vi "GetLastChar.vi"(10 "String":string) -> (2 "String 2":string)   [LabVIEW 2016]
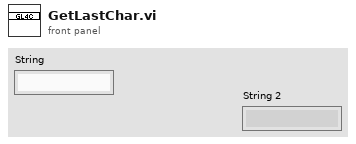
[diagram p1: front panel]
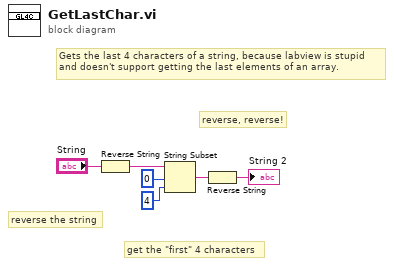
[diagram p0: block diagram]
diagram:
  # "reverse, reverse!"
  # "get the \"first\" 4 characters"
  # "reverse the string"
  # "Gets the last 4 characters of a string, because labview is stupid\nand doesn't support getting the last elements of an array."
  n1 = Reverse String(1:"String") -> (0:w4:string)
  n2 = String Subset(string=w4, offset (0)=0, length (rest)=4 ("length (rest)")) -> (substring=w3:string)
  n3 = Reverse String(1:w3) -> (0:→"String 2":string)
